vi "Configure Surge-Drop Voltage.vi"(0 "VISA resource name":refnum<visa-resource-name>, 5 "Surge Drop Voltage (100 V)":dbl=100.0 min=0.0 max=300.0 format="%#.1f", 11 "error in (no error)":errorcluster) -> (4 "VISA resource name out":refnum<visa-resource-name>, 15 "error out":errorcluster)   [LabVIEW 2020, in "eec 6700.lvlib"]
doc: "Sets the <B>Surge-Drop Voltage</B> of the power source instrument.\n\n<B>Range</B> : 0.0~300.0 V\n\nThe Surge-Drop Volt parameter setting configures a surge or drop in the voltage output. Whether the voltage is a surge or a drop depends on the voltage that is programmed for this parameter. For example if the output voltage is programmed at 120 volts and the operator programs in a Surge Drop-Volt of 150 volts this would be a surge of 30 volts. The opposite holds true; if the Surge Drop-Volt is programmed at 90 volts this would be a drop of 30 volts."
uses:
  <instrlib>/EEC6700LV-driver/eec 6700.lvlib
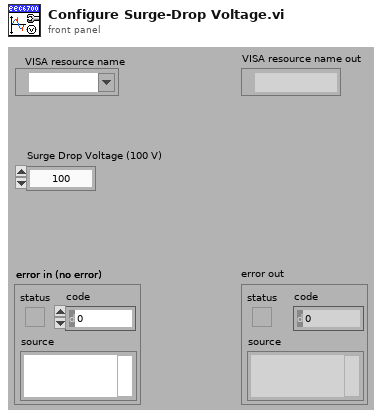
[diagram p1: front panel]
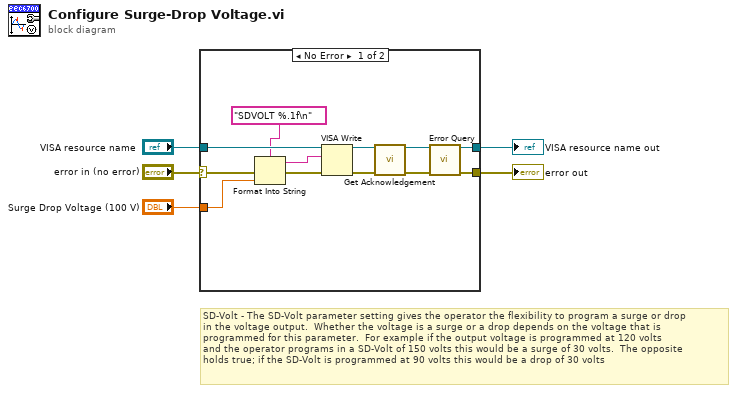
[diagram p0: block diagram]
diagram:
  # "SD-Volt - The SD-Volt parameter setting gives the operator the flexibility to program a surge or drop\nin the voltage output.  Whether the voltage is a surge or a drop depends on the voltage that is\nprogrammed for this parameter.  For example if the output voltage is programmed at 120 volts \nand the operator programs in a SD-Volt of 150 volts this would be a surge of 30 volts.  The opposite \nholds true; if the SD-Volt is programmed at 90 volts this would be a drop of 30 volts"
  n1 = case shown="No Error" "error in (no error)" {
    selector: "error in (no error)" -> [w11 w19]
    tunnel: "VISA resource name" -> [w17 w18]
    tunnel: [w14 w18] -> w4
    tunnel: [w13 w19] -> w3
    tunnel: "Surge Drop Voltage (100 V)" -> [w12 _]
    frame No Error {
      n2 = Format Into String(format string="SDVOLT %.1f\n" ("Command"), error in=w11, w12) -> (resulting string=w15:string, error out=w10:errorcluster)  [unwired: 1 in]
      n3 = VISA Write(VISA resource name=w17, write buffer=w15, error in (no error)=w10) -> (VISA resource name out=w7:refnum<visa-resource-name>, error out=w6:errorcluster)  [unwired: 1 out]
      n4 = call <instrlib>:"Get Acknowledgement.vi"("VISA resource name"=w7, "error in (no error)"=w6) -> ("VISA resource name out"=w8:refnum<visa-resource-name>, "error out"=w9:errorcluster)  [unwired: 12 in]
      n5 = call <instrlib>:"Error Query.vi"("VISA resource name"=w8, "error in (no error)"=w9) -> ("VISA resource name out"=w14:refnum<visa-resource-name>, "error out"=w13:errorcluster)  [unwired: 10 in, 2 out]
    }
    frame Error {
    }
  }
  "error out" <- w3
  "VISA resource name out" <- w4
